vi "Test User Input In Focus on Depositing.vi"(8 "error in (no error)":errorcluster, 11 "Test Case In":refnum<class "View Model Test.lvclass">) -> (0 "error out":errorcluster, 3 "Test Case Out":refnum<class "View Model Test.lvclass">)   [LabVIEW 2020, in "View Model Test.lvclass"]
uses:
  View Model Test.lvclass
  C:/Program Files (x86)/National Instruments/LabVIEW 2020/vi.lib/Astemes/LUnit/Test Case.lvclass
  ATM View Model/Controls.ctl
  ATM Controller/State.ctl
  <vilib>/Astemes/LUnit/Test Case.lvclass/Test Case.ctl
  <vilib>/Astemes/LUnit/Palette/Fail.vi
  <vilib>/Astemes/LUnit/Palette/Pass.vi
  <vilib>/Astemes/LUnit/Set Assertion Type.vi
  <vilib>/Astemes/LUnit/Add test result.vi
  <vilib>/Astemes/LUnit/LUnit Record Assertion Result.vi
  <vilib>/Astemes/LUnit/LUnit Aggregate Assertion Results.vi
  <vilib>/Astemes/LUnit/Method Result/LUnit Merge Status.vi
  <vilib>/Astemes/LUnit/LUnit Concatenate result strings.vi
  View Model Test.lvclass/View Model Test.ctl
  ATM View Model/ATM View Model.lvclass
  ATM Controller/ATM Controller.lvclass
  <vilib>/Astemes/LUnit/Test Case.lvclass
  C:/git/astemes-tdd-cld/source/Tests/Start Application Run Test/View Model Test.lvclass
panel:
  in  "Test Control":string
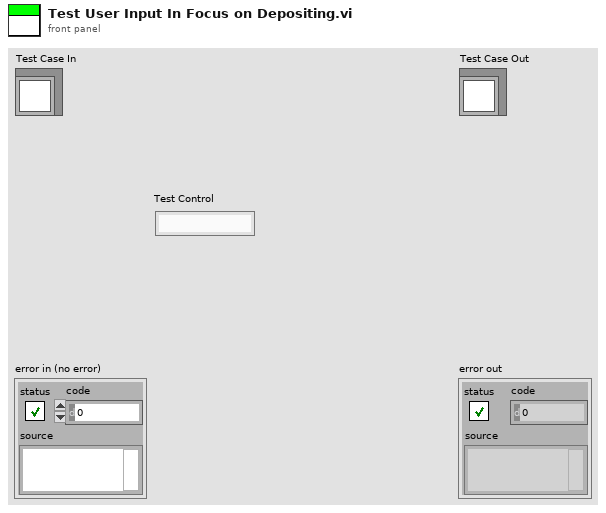
[diagram p1: front panel]
types:
  T1 = enum32{"Invalid", "Standard", "Closed", "Hidden", "Minimized", "Maximized"}
  T2 = typedef "ATM Controller.lvclass/State.ctl" = enum16{"Start", "Card Inserted", "Verification Failed", "Verification Succeeded", "Depositing", "Depositing Completed", "Withdrawing", "Terminate"}
  T3 = typedef "ATM View Model.lvclass/Controls.ctl" = enum16{"User Input", "Enter", "Left Menu", "Right Menu", "Left Button", "Right Button", "Card Simulator"}
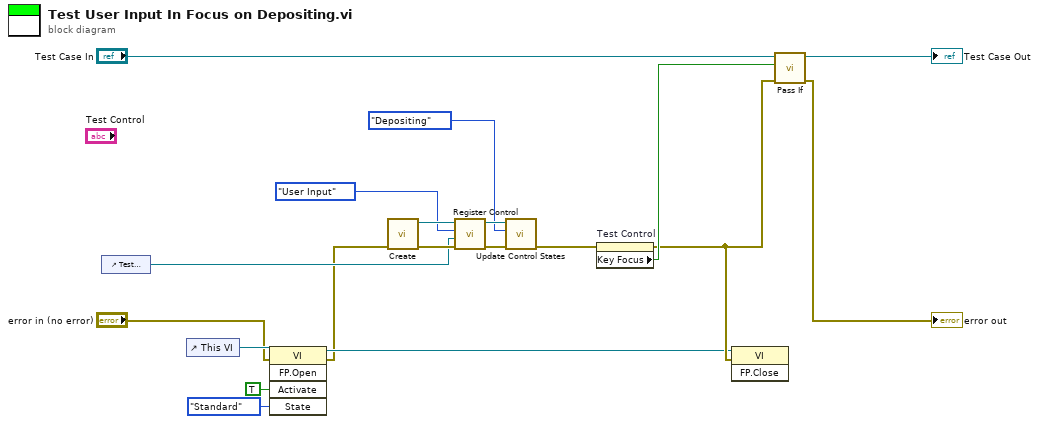
[diagram p0: block diagram]
diagram:
  n1 = control-ref of="Test Control"() -> (w12:refnum<vi>)
  n2 = control-ref of="This VI"() -> (w7:refnum<vi>)
  n3 = invoke class="VI" method="FP.Open"(reference=w7, error in="error in (no error)", "Activate"=TRUE ("Activate?"), "State"=T1."Standard") -> (reference out=w3:refnum<vi>, error out=w1:errorcluster)  [unwired: 1 in, 3 out]
  n4 = call "Create.vi"("error in (no error)"=w1) -> ("error out"=w15:errorcluster, "ATM View Model out"=w16:refnum<class "ATM View Model.lvclass">)  [unwired: 9 in]
  n5 = call "Register Control.vi"("error in (no error)"=w15, "Control ref"=w12, "Control"=Controls."User Input" ("Controls"), "ATM View Model in"=w16) -> ("error out"=w13:errorcluster, "ATM View Model out"=w14:refnum<class "ATM View Model.lvclass">)  [unwired: 6 in]
  n6 = call "Update Control States.vi"("error in (no error)"=w13, "ATM State"=State."Depositing", "ATM View Model In"=w14) -> ("error out"=w10:errorcluster)  [unwired: 7 in, 1 out]
  n7 = property on="Test Control" class="Str"(error in=w10) -> (error out=w4:errorcluster, "Key Focus"=w9:bool)  [unwired: 1 in, 1 out]
  n8 = invoke class="VI" method="FP.Close"(reference=w3, error in=w4) -> ()  [unwired: 1 in, 3 out]
  n9 = call <vilib>:"Pass If.vi"("error in (no error)"=w4, "Pass?"=w9, "LUnit Test Case In"="Test Case In") -> ("error out"=→"error out":errorcluster, "LUnit Test Case Out"=→"Test Case Out":refnum<class "View Model Test.lvclass">)  [unwired: 7 in]
